vi "scan2d_writes_scan_settings.vi"(8 "error in (no error)":errorcluster, 10 "scan-2d-settings":T1, 11 "scan_2d in":refnum<class "scan_2d.lvclass">) -> (0 "error out":errorcluster, 3 "scan_2d out":refnum<class "scan_2d.lvclass">)   [LabVIEW 2015, in "scan_2d.lvclass"]
uses:
  scan_2d.lvclass
  scan_2d_settings.ctl
  Scan/scan_record.ctl
  scan_2d_stage_settings.ctl
  scan_2d.lvclass/scan_2d.ctl
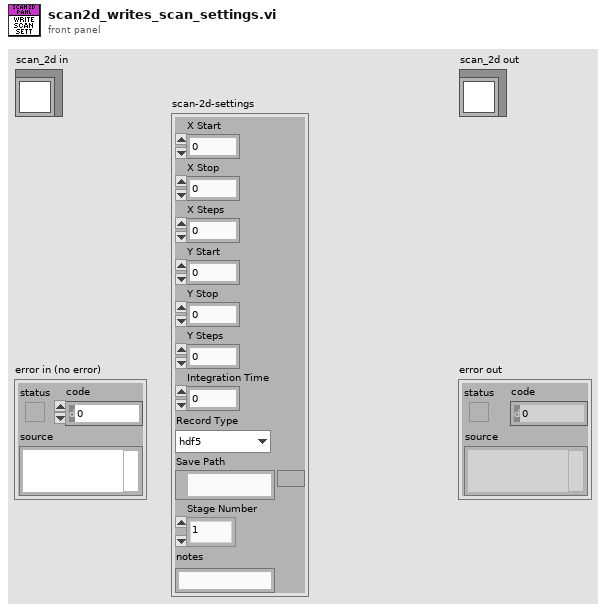
[diagram p1: front panel]
types:
  T1 = typedef "scan_2d_settings.ctl" = cluster{"X Start":dbl, "X Stop":dbl, "X Steps":u32, "Y Start":dbl, "Y Stop":dbl, "Y Steps":u32, "Integration Time":dbl, "Record Type":T2, "Save Path":path, "Stage Number":enum16{"1", "2"}, "notes":string}
  T2 = typedef "scan_record.ctl" = enum16{"hdf5", "legacy", "None"}
  T3 = typedef "scan_2d_stage_settings.ctl" = cluster{"X Start":dbl, "X Stop":dbl, "X Steps":u32, "Y Start":dbl, "Y Stop":dbl, "Y Steps":u32}
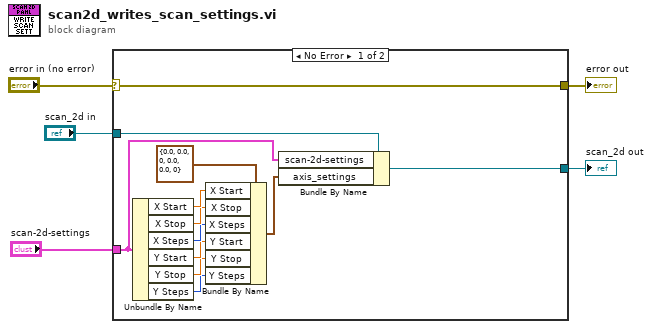
[diagram p0: block diagram]
diagram:
  n1 = case shown="No Error" "error in (no error)" {
    selector: "error in (no error)" -> [w17 w19]
    tunnel: [w17 w19] -> w4
    tunnel: [w15 w18] -> w2
    tunnel: "scan_2d in" -> [w16 w18]
    tunnel: "scan-2d-settings" -> [w6 _]
    frame No Error {
      n2 = Unbundle By Name(w6) -> ("X Start"=w13:dbl, "X Stop"=w12:dbl, "X Steps"=w11:u32, "Y Start"=w10:dbl, "Y Stop"=w9:dbl, "Y Steps"=w8:u32)
      n3 = Bundle By Name(cluster=T3 {"X Start"=0.0, "X Stop"=0.0, "X Steps"=0, "Y Start"=0.0, "Y Stop"=0.0, "Y Steps"=0} ("scan-settings"), "X Start"=w13, "X Stop"=w12, "X Steps"=w11, "Y Start"=w10, "Y Stop"=w9, "Y Steps"=w8) -> (w7:T3)
      n4 = Bundle By Name(cluster=w16, "scan-2d-settings"=w6, "axis_settings"=w7) -> (w15:refnum<class "scan_2d.lvclass">)
    }
    frame Error {
    }
  }
  "error out" <- w4
  "scan_2d out" <- w2
